vi "Matrix_Exp.vi"(11 "input matrix":T1) -> (0 "Error":bool, 3 "output matrix":T1)   [LabVIEW 2019, in "Trajectory_Library.lvlib"]
doc: "Computes the matrix exponential using Eigen's solver. This method only works for square matrices, and will otherwise throw an MatrixDimensionException.\n \nInputs:\n - input matrix -- The input matrix\n\nOutputs:\n - output matrix -- The exponential of A.\n - error -- If TRUE, an error occured."
uses:
  Trajectory_Library.lvlib
  <vilib>/Analysis/Matrix/Datatypes/RealMatrix.ctl
  <vilib>/Analysis/7linalg.llb/Real Matrix Exp.vi
  <vilib>/Analysis/NI_AALBase.lvlib
  <vilib>/Analysis/Matrix/NI_Matrix.lvlib
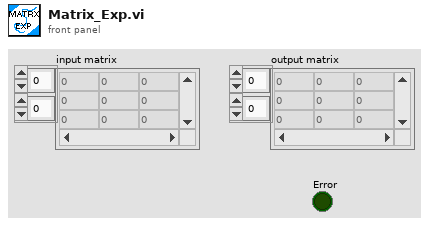
[diagram p1: front panel]
types:
  T1 = typedef "NI_Matrix.lvlib/RealMatrix.ctl" = dbl[][]
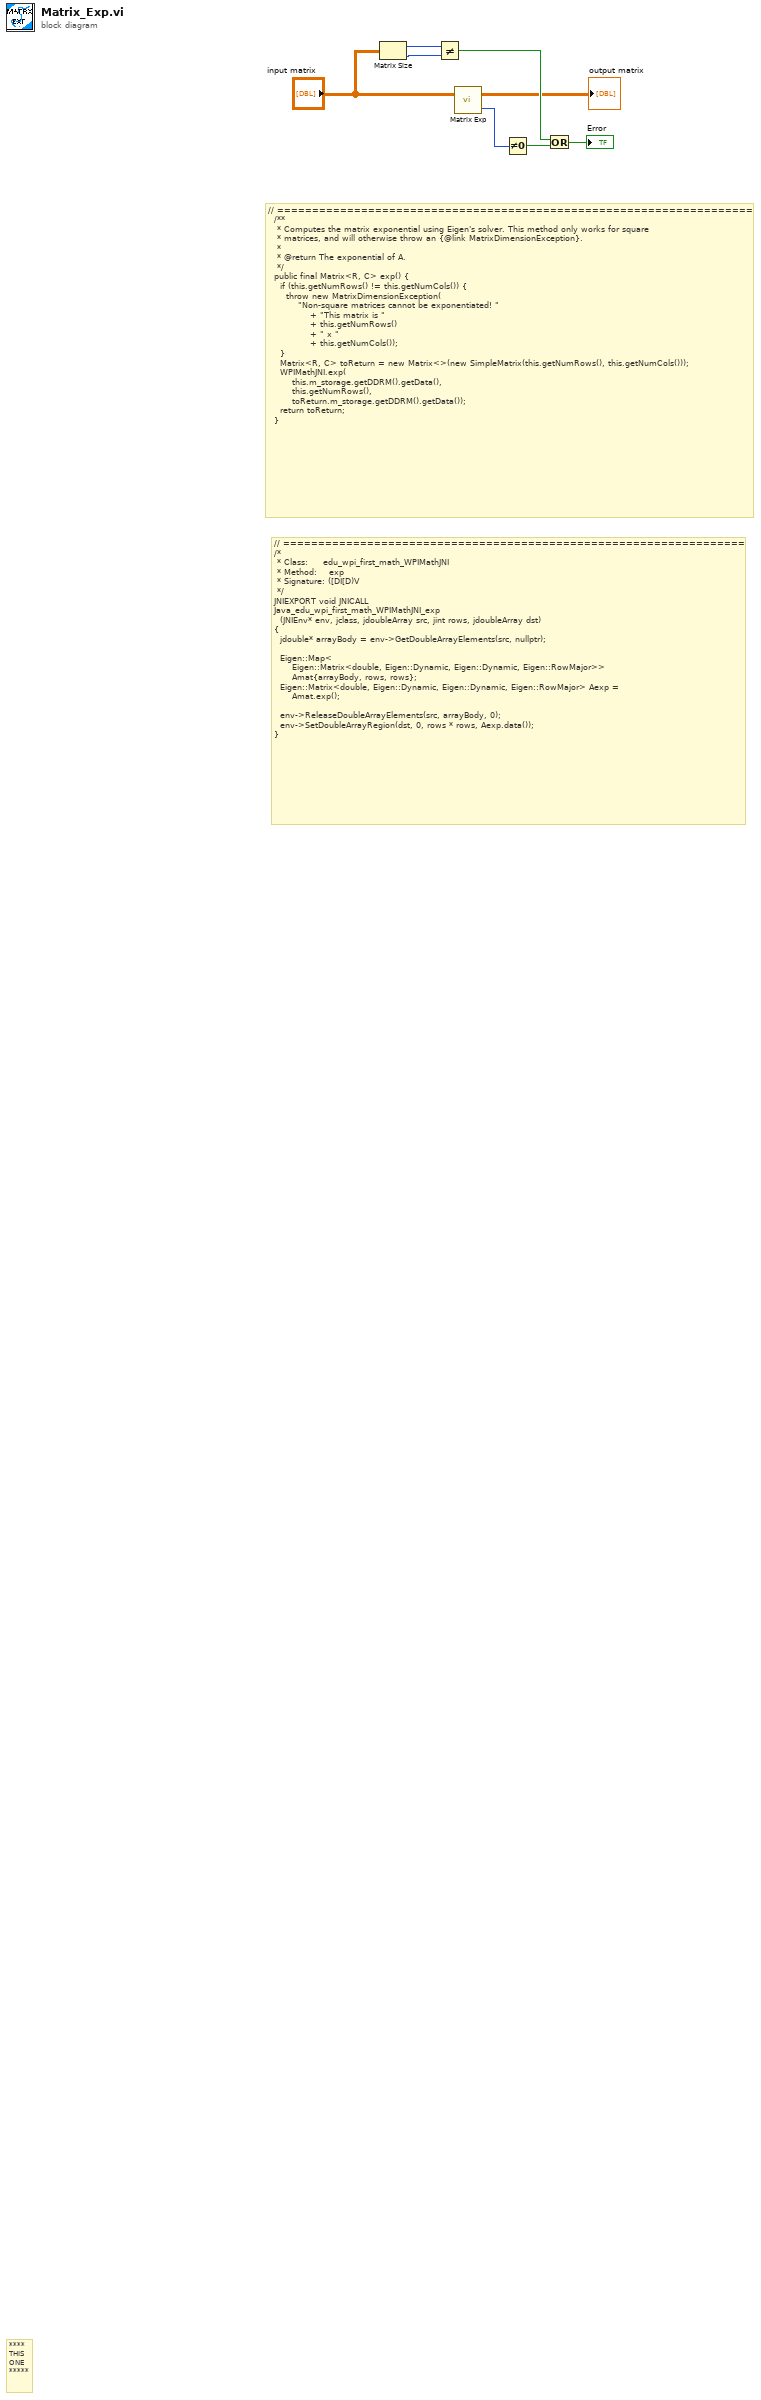
[diagram p0: block diagram]
diagram:
  # "// ==================================================================\n/*\n * Class:     edu_wpi_first_math_WPIMathJNI\n * Method:    exp\n * Signature: ([DI[D)V\n */\nJNIEXPORT void JNICALL\nJava_edu_wpi_first_math_WPIMathJNI_exp\n  (JNIEnv* env, jclass, jdoubleArray src, jint rows, jdoubleArray dst)\n{\n  jdouble* arrayBody = env->GetDoubleArrayElements(src, nullptr);\n\n  Eigen::Map<\n      Eigen::Matrix<double, Eigen::Dynamic, Eigen::Dynamic, Eigen::RowMajor>>\n      Amat{arrayBody, rows, rows};\n  Eigen::Matrix<double, Eigen::Dynamic, Eigen::Dynamic, Eigen::RowMajor> Aexp =\n      Amat.exp();\n\n  env->ReleaseDoubleArrayElements(src, arrayBody, 0);\n  env->SetDoubleArrayRegion(dst, 0, rows * rows, Aexp.data());\n}"
  # "// ====================================================================\n  /**\n   * Computes the matrix exponential using Eigen's solver. This method only works for square\n   * matrices, and will otherwise throw an {@link MatrixDimensionException}.\n   *\n   * @return The exponential of A.\n   */\n  public final Matrix<R, C> exp() {\n    if (this.getNumRows() != this.getNumCols()) {\n      throw new MatrixDimensionException(\n          \"Non-square matrices cannot be exponentiated! \"\n              + \"This matrix is \"\n              + this.getNumRows()\n              + \" x \"\n              + this.getNumCols());\n    }\n    Matrix<R, C> toReturn = new Matrix<>(new SimpleMatrix(this.getNumRows(), this.getNumCols()));\n    WPIMathJNI.exp(\n        this.m_storage.getDDRM().getData(),\n        this.getNumRows(),\n        toReturn.m_storage.getDDRM().getData());\n    return toReturn;\n  }"
  # "****\nTHIS\nONE\n*****"
  n1 = Matrix Size(0:"input matrix") -> (1:w8:i32, 2:w7:i32)
  n2 = Not Equal?(x=w8, y=w7) -> (x != y?=w4:bool)
  n3 = call-poly <vilib>:"Matrix Exp.vi"("Input Matrix"="input matrix") -> ("error"=w1:i32, "Matrix Exp"=→"output matrix":T1)  [unwired: 1 in]
  n4 = Not Equal To 0?(x=w1) -> (x != 0?=w5:bool)
  n5 = Or(x=w4, y=w5) -> (x .or. y?=→"Error":bool)
